vi "ColorProcessing2016_Custom.vi"(5 "LED Color Ref":refnum<vi>, 7 "Image Ctl Refnum":refnum<vi>, 9 "LED Color":T6={"Hue"={62.82225036621094, 124.95552062988281}, "Sat"={13.666671752929688, 253.6666717529297}, "Val"={150.51114654541016, 255.0}} {"Hue" scale=0.0..255.0 scale format="%#_3g"}, 10 "Mask":T5=refnum, 11 "Original":T5=refnum) -> (0 "Blob array":T2(array[cluster])=[{"Area"=410.0, "Object Info"={"Object Center"={"X"=155.50975, "Y"=158.86829}, "Bounding Box"={"X Left"=142, "Y Top"=150, "X Right"=169, "Y Bottom"=168}, "Area"=410.0, "Orientation"=9.943739, "Aspect Ratio"=1.5, "Nb Holes"=0}}], 1 "Masked":T5(plugin-control), 2 "Targets":T4[](array[typedef]), 3 "Original Image":T5(plugin-control), 4 "Scored Particle Info 2":T1(array[cluster]))   [LabVIEW 2015]
uses:
  Camera Types.ctl
  <vilib>/vision/Image Controls.llb/IMAQ Image.ctl
  Scores.ctl
  <vilib>/vision/NI_Vision_Development_Module.lvlib
panel:
  in  "Particle Count Limit":i32=3
  out "Scored Particle Info":T1(array[cluster])
  in  "Area Size Limit %":dbl=0.5
  in  "Settings":T3={"Objects"=0, "Threshold"=1, "Reject Border"=TRUE, "Fill Holes"=FALSE, "Min Object Size"=TRUE, "Min Size"=350, "Max Object Size"=TRUE, "Max Size"=700, "Show Search Area"=TRUE, "Show Center"=TRUE, "Show Bounding Box"=TRUE} {"Objects" items=["Bright Objects", "Dark Objects"]; "Threshold" min=1 max=999999999 step=1; "Max Size" min=1 max=999999999 step=1; "Min Size" min=1 max=999999999 step=1}
  out "Qualified Particles":i32=3
  out "Sorted Particle Scores":T7(array[cluster]) {"Center" format="%#_3g"; "Moment Factor" format="%#_3g"; "Aspect Ratio" format="%#_3g"; "Area to CH" format="%#_3g"; "X" format="%#_3g"; "Y" format="%#_3g"}
  out "Detected Targets":T8(array[cluster]) {"Normalized Rect"."Numeric 5" format="%#_2g"; "Normalized Rect"."Numeric 3" format="%#_2g"; "Normalized Rect"."Numeric 2" format="%#_2g"; "Normalized Rect"."Numeric" format="%#_2g"}
  in  "Aspect Ratio Fudge Factor":dbl=1.0
  out "Highest Avg Score":dbl=85.32840563115018 format="%#_3g"
  in  "Min Score Threshold":i32=70
  in  "Camera Type":T9=enum."MS HD3000 square"
  in  "Emphasize Limit Tests":bool=TRUE
  in  "Std Devs for Calibration":cluster{"H":dbl, "S":dbl, "V":dbl}={"H"=4.0, "S"=6.0, "V"=6.0}
  # "Density Profile"
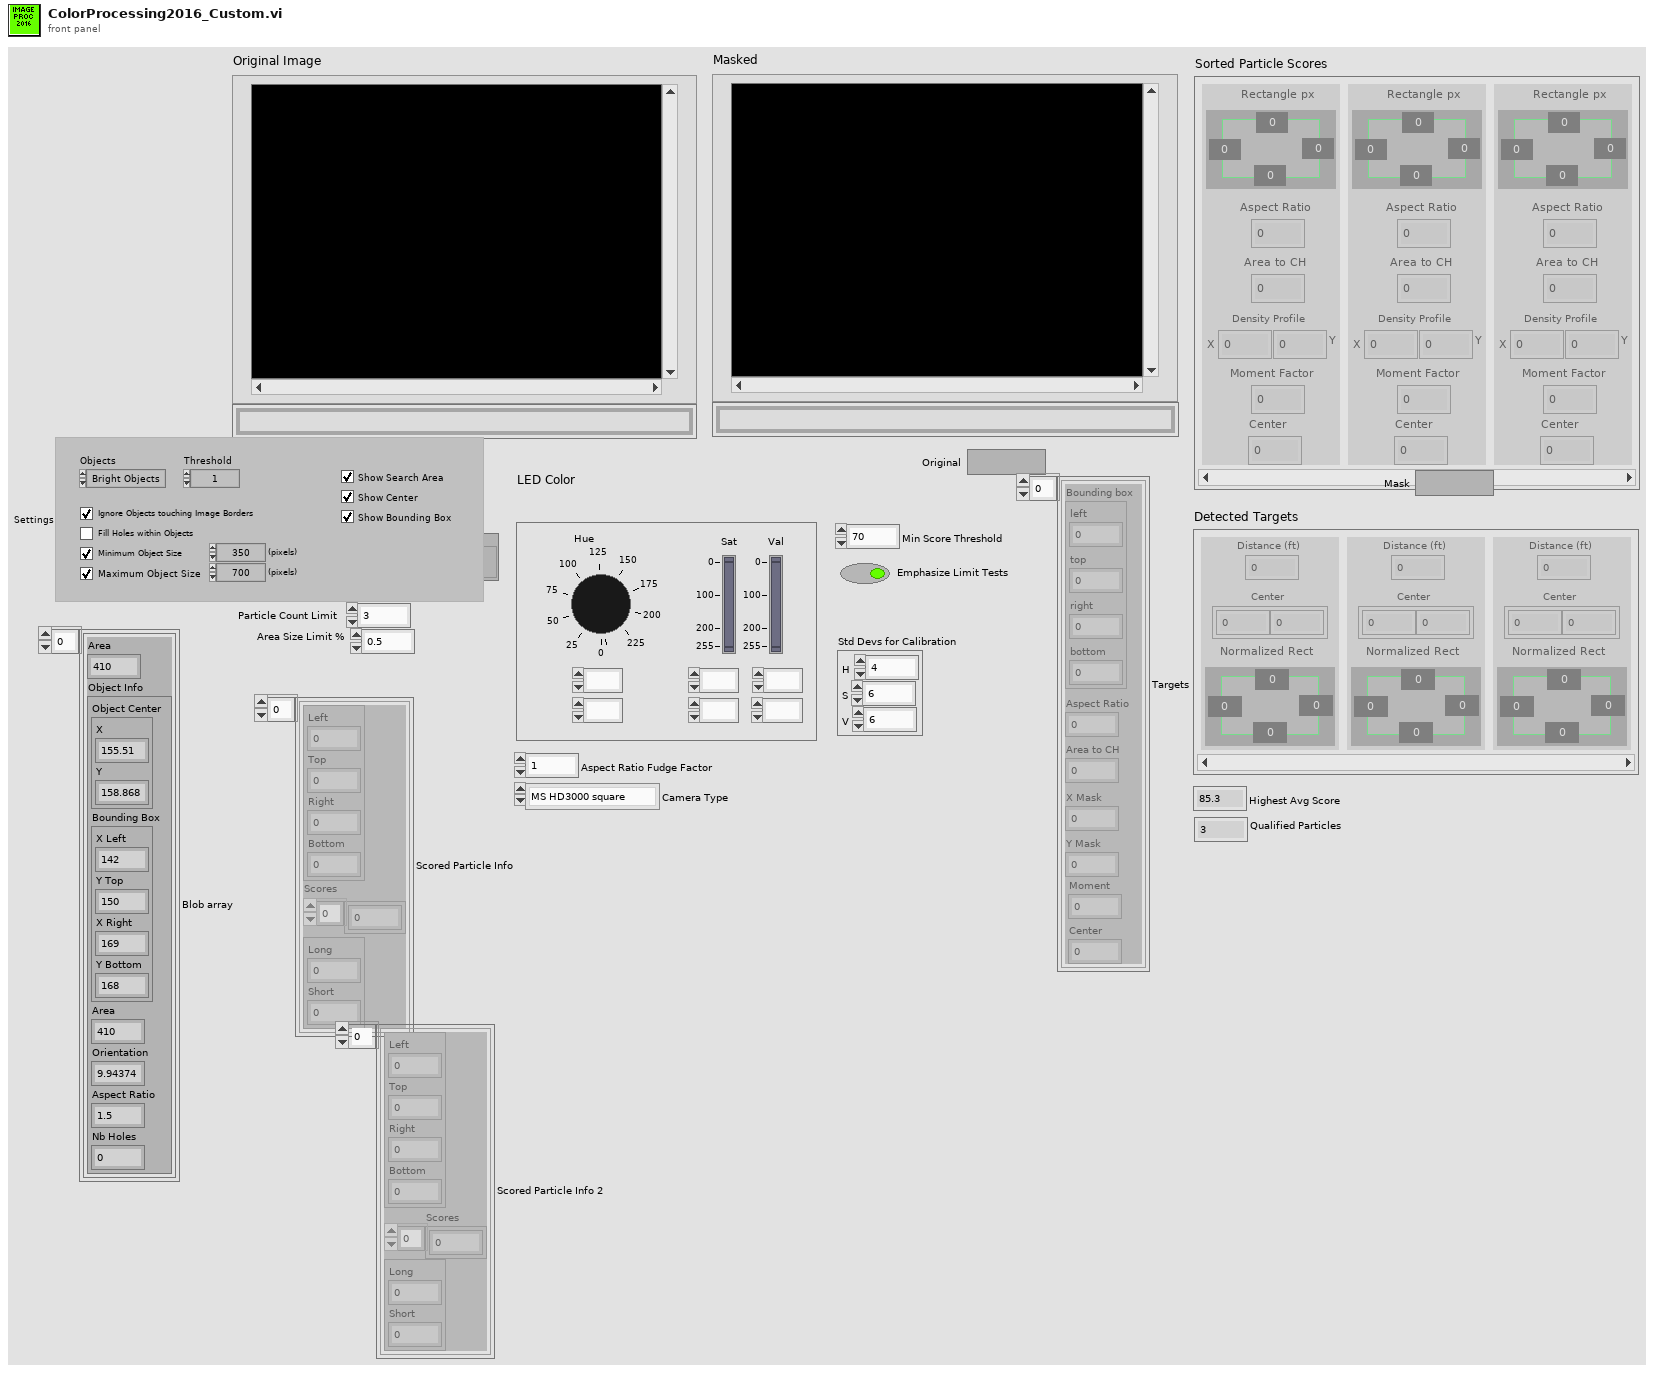
[diagram p1: front panel]
types:
  T1 = cluster{cluster{"Left":dbl, "Top":dbl, "Right":dbl, "Bottom":dbl}, "Scores":dbl[], cluster{"Long":dbl, "Short":dbl}}[]
  T2 = cluster{"Area":sgl, "Object Info":cluster{"Object Center":cluster{"X":sgl, "Y":sgl}, "Bounding Box":cluster{"X Left":i32, "Y Top":i32, "X Right":i32, "Y Bottom":i32}, "Area":sgl, "Orientation":sgl, "Aspect Ratio":sgl, "Nb Holes":i32}}[]
  T3 = cluster{"Objects":u16, "Threshold":i32, "Reject Border":bool, "Fill Holes":bool, "Min Object Size":bool, "Min Size":i32, "Max Object Size":bool, "Max Size":i32, "Show Search Area":bool, "Show Center":bool, "Show Bounding Box":bool}
  T4 = typedef "Scores.ctl" = cluster{"Bounding box":cluster{"left":dbl, "top":dbl, "right":dbl, "bottom":dbl}, "Aspect Ratio":dbl, "Area to CH":dbl, "X Mask":dbl, "Y Mask":dbl, "Moment":dbl, "Center":dbl}
  T5 = typedef "IMAQ Image.ctl" = refnum<image>
  T6 = cluster{"Hue":cluster{dbl, dbl}, "Sat":cluster{dbl, dbl}, "Val":cluster{dbl, dbl}}
  T7 = cluster{"Rectangle px":cluster{"Numeric":dbl, "Numeric 2":dbl, "Numeric 3":dbl, "Numeric 5":dbl}, "Aspect Ratio":dbl, "Area to CH":dbl, "X":dbl, "Y":dbl, "Moment Factor":dbl, "Center":dbl}[]
  T8 = cluster{"Distance (ft)":dbl, "Center":cluster{dbl, dbl}, "Normalized Rect":cluster{"Numeric":dbl, "Numeric 2":dbl, "Numeric 3":dbl, "Numeric 5":dbl}}[]
  T9 = typedef "Camera Types.ctl" = enum16{"206", "1011", "1013", "MS HD3000 square", "MS HD3000 640x480"}
  T10 = typedef "Particle Parameters" = i32
  T11 = typedef "IMAQ Rectangle" = cluster{"Left":i32, "Top":i32, "Right":i32, "Bottom":i32, "Rotation":dbl}
  T12 = typedef "Image Type" = u32
  T13 = cluster{"Object Center":cluster{"X":sgl, "Y":sgl}, "Bounding Box":cluster{"X Left":i32, "Y Top":i32, "X Right":i32, "Y Bottom":i32}, "Area":sgl, "Orientation":sgl, "Aspect Ratio":sgl, "Nb Holes":i32}[]
  T14 = cluster{"Area":sgl, "Object Info":cluster{"Object Center":cluster{"X":sgl, "Y":sgl}, "Bounding Box":cluster{"X Left":i32, "Y Top":i32, "X Right":i32, "Y Bottom":i32}, "Area":sgl, "Orientation":sgl, "Aspect Ratio":sgl, "Nb Holes":i32}}
  T15 = cluster{"Rectangle":cluster{"Numeric":dbl, "Numeric 2":dbl, "Numeric 3":dbl, "Numeric 5":dbl}, "L":dbl, "Area to CH":dbl, "X":dbl, "Y":dbl, "Moment Factor":dbl, "Center":dbl}[]
  T16 = cluster{cluster{dbl, dbl}, cluster{dbl, dbl}, cluster{dbl, dbl}}
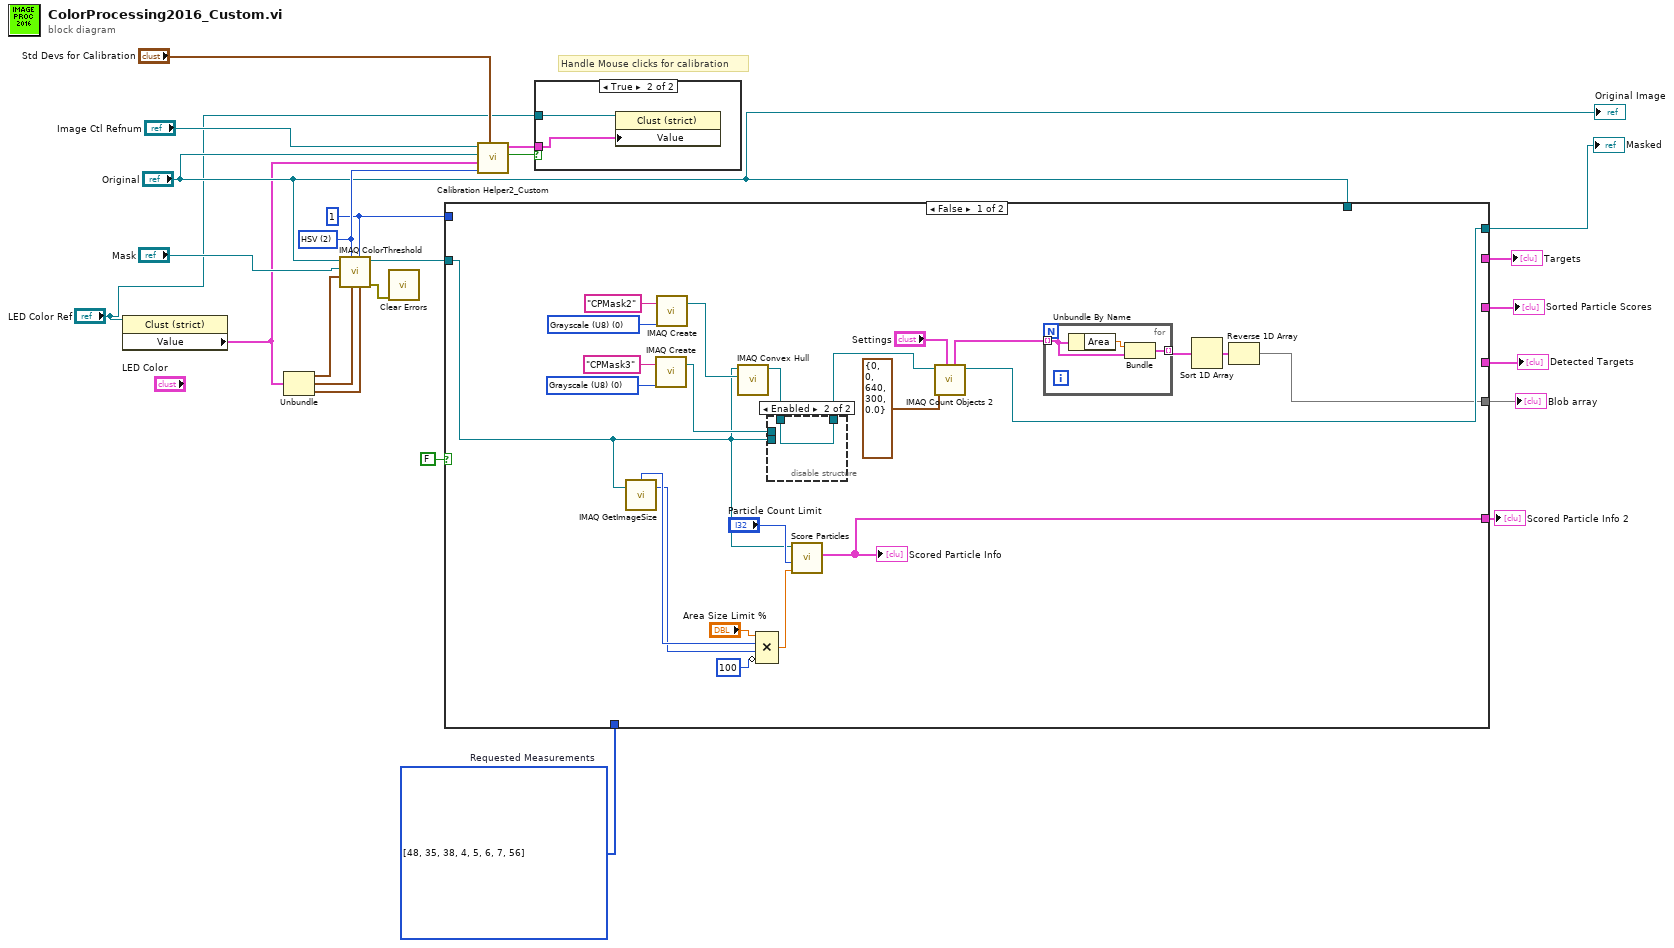
[diagram p0: block diagram]
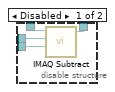
[diagram p2: hidden frame]
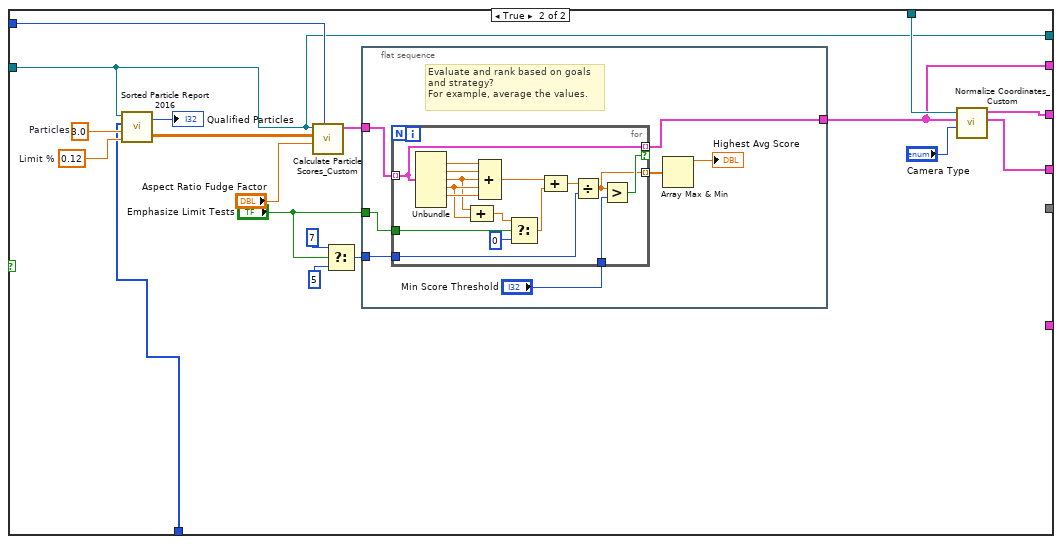
[diagram p3: hidden frame]
diagram:
  w2 = T10[] [48, 35, 38, 4, 5, 6, 7, 56] items=["Center of Mass X", "Center of Mass Y", "First Pixel X", "First Pixel Y", "Bounding Rect Left", "Bounding Rect Top", "Bounding Rect Right", "Bounding Rect Bottom", "Max Feret Diameter Start X", "Max Feret Diameter Start Y", "Max Feret Diameter End X", "Max Feret Diameter End Y", "Max Horiz. Segment Length Left", "Max Horiz. Segment Length Right", "Max Horiz. Segment Length Row", "-", "Bounding Rect Width", "Bounding Rect Height", "Bounding Rect Diagonal", "Perimeter", "Convex Hull Perimeter", "Holes' Perimeter", "Max Feret Diameter", "Equivalent Ellipse Major Axis", "Equivalent Ellipse Minor Axis", "Equivalent Ellipse Minor Axis (Feret)", "Equivalent Rect Long Side", "Equivalent Rect Short Side", "Equivalent Rect Diagonal", "Equivalent Rect Short Side (Feret)", "Average Horiz. Segment Length", "Average Vert. Segment Length", "Hydraulic Radius", "Waddel Disk Diameter", "-", "Area", "Holes' Area", "Particle & Holes' Area", "Convex Hull Area", "Image Area", "-", "Number of Holes", "Number of Horiz. Segments", "Number of Vert. Segments", "-", "Orientation", "Max Feret Diameter Orientation", "-", "% Area/Image Area", "% Area/(Particle & Holes' Area)", "Ratio of Equivalent Ellipse Axes", "Ratio of Equivalent Rect Sides", "-", "Elongation Factor", "Compactness Factor", "Heywood Circularity Factor", "Type Factor", "-", "Sum X", "Sum Y", "Sum XX", "Sum XY", "Sum YY", "Sum XXX", "Sum XXY", "Sum XYY", "Sum YYY", "-", "Moment of Inertia XX", "Moment of Inertia XY", "Moment of Inertia YY", "Moment of Inertia XXX", "Moment of Inertia XXY", "Moment of Inertia XYY", "Moment of Inertia YYY", "Norm. Moment of Inertia XX", "Norm. Moment of Inertia XY", "Norm. Moment of Inertia YY", "Norm. Moment of Inertia XXX", "Norm. Moment of Inertia XXY", "Norm. Moment of Inertia XYY", "Norm. Moment of Inertia YYY", "Hu Moment 1", "Hu Moment 2", "Hu Moment 3", "Hu Moment 4", "Hu Moment 5", "Hu Moment 6", "Hu Moment 7"]  # Requested Measurements
  w17 = 1 ("Replace Value")
  w22 = u16 2 items=["RGB", "HSL", "HSV", "HSI"] ("Color Mode")
  # "Handle Mouse clicks for calibration"
  n1 = property class="Clust (strict)"(reference="LED Color Ref") -> ("Value"=w8:T6)  [unwired: 1 in, 2 out]
  n2 = Unbundle(w8) -> ("Hue"=w14:cluster{dbl, dbl}, "Sat"=w15:cluster{dbl, dbl}, "Val"=w16:cluster{dbl, dbl})
  n3 = call "IMAQ ColorThreshold"("Blue or Luma or Val or Inten Range"=w16, "Replace Value"=w17, "Green or Sat Range"=w15, "Color Mode"=w22, "Red or Hue Range"=w14, "Image Dst"="Mask", "Image Src"="Original") -> ("error out"=w19:errorcluster, "Image Dst Out"=w6:T5)  [unwired: 3 in]
  n4 = call <vilib>:"Clear Errors.vi"("error in (no error)"=w19) -> ()  [unwired: 5 in, 2 out]
  n5 = case shown="False" FALSE {
    tunnel: [_ w65] -> w18
    tunnel: w17 -> [_ w64]
    tunnel: "Original" -> [_ w59]
    tunnel: [_ w58] -> w10
    tunnel: [_ w57] -> w9
    tunnel: w6 -> [w26 w56]
    tunnel: [w35 w56] -> w5
    tunnel: [w34 _] -> w4
    tunnel: w2 -> [_ w55]
    tunnel: [w27 _] -> w1
    frame False {
      w41 = T12 0 items=["Grayscale (U8)", "Grayscale (I16)", "Grayscale (SGL)", "Complex (CSG)", "RGB (U32)", "HSL (U32)", "RGB (U64)", "Grayscale (U16)"] ("Image Type")
      w39 = T12 0 items=["Grayscale (U8)", "Grayscale (I16)", "Grayscale (SGL)", "Complex (CSG)", "RGB (U32)", "HSL (U32)", "RGB (U64)", "Grayscale (U16)"] ("Image Type")
      n6 = call "IMAQ GetImageSize"("Image"=w26) -> ("Y Resolution"=w24:i32, "X Resolution"=w25:i32)  [unwired: 3 in, 1 out]
      n7 = call "IMAQ Create"("Image Name"="CPMask3", "Image Type"=w41) -> ("New Image"=w43:T5)  [unwired: 2 in, 2 out]
      n8 = call "IMAQ Create"("Image Name"="CPMask2", "Image Type"=w39) -> ("New Image"=w40:T5)  [unwired: 2 in, 2 out]
      n9 = call "IMAQ Convex Hull"("Image Dst"=w40, "Image Src"=w26) -> ("Image Dst Out"=w33:T5)  [unwired: 8 in, 1 out]
      n10 = Compound Arithmetic op=MULTIPLY("Area Size Limit %", w25, w24, invert 100 ("length")) -> (w28:dbl)
      n11 = disable-structure shown="Enabled" {
        disable-tunnel: w43 -> [w50 _]
        disable-tunnel: w26 -> [w49 _]
        disable-tunnel: w33 -> [w48 w51]
        disable-tunnel: [w47 w51] -> w32
        frame Disabled {
          n12 = call "IMAQ Subtract"("Image Src A"=w48, "Image Dst"=w50, "Image Src B"=w49) -> ("Image Dst Out"=w47:T5)  [unwired: 4 in, 1 out]
        }
        frame Enabled {
        }
      }
      n13 = call "Score Particles.vi"("Area Size Limit"=w28, "Particle Count Limit"="Particle Count Limit", "Image Refnum in"=w26) -> ("Scored Particle Info"=w27:T1)  [unwired: 7 in, 1 out]
      "Scored Particle Info" <- w27
      n14 = call "IMAQ Count Objects 2"("Settings"="Settings", "Search Rect (entire image)"=T11 {"Left"=0, "Top"=0, "Right"=640, "Bottom"=300, "Rotation"=0.0}, "Image"=w32) -> ("Image Out"=w35:T5, "Objects"=w44:T13)  [unwired: 4 in, 3 out]
      n15 = for {
        tunnel: w44 -> [w54] mode=indexing
        tunnel: [w52] -> w45 mode=indexing
        n16 = Unbundle By Name(w54) -> ("Area"=w53:sgl)
        n17 = Bundle("Area"=w53, "Object Info"=w54) -> (w52:T14)  [unwired: 1 in]
      }
      n18 = Sort 1D Array(array=w45) -> (sorted array=w46:T2)
      n19 = Reverse 1D Array(array=w46) -> (reversed array=w34:T2)
    }
    frame True {
      w63 = 0.12  # Limit %
      w60 = 3.0  # Particles
      n20 = call "Sorted Particle Report 2016.vi"("Min Area Size %"=w63, "Particle Count Limit"=w60, "Pixel Measurements"=w55, "Image in"=w56) -> ("Sorted Data"=w62:dbl[][], "Particles"=→"Qualified Particles":i32)
      n21 = call "Calculate Particle Scores_Custom.vi"("Pixel Value"=w64, "Aspect Fudge Factor"="Aspect Ratio Fudge Factor", "Sorted Data"=w62, "Image in"=w56) -> ("Scores"=w67:T4[])  [unwired: 7 in]
      n22 = Select(t=7, s="Emphasize Limit Tests", f=5) -> (s? t:f=w71:i32)
      n23 = flat-sequence {
        tunnel: w67 -> [w78]
        tunnel: [w79] -> w58
        tunnel: w71 -> [w75]
        tunnel: "Emphasize Limit Tests" -> [w73]
        frame #0 {
          # "Evaluate and rank based on goals\nand strategy?\nFor example, average the values."
          n24 = for {
            tunnel: w78 -> [w93] mode=indexing
            tunnel: [w93] -> w79 mode=indexing if=w92
            tunnel: [w91] -> w77 mode=indexing
            tunnel: w75 -> [w90]
            tunnel: "Min Score Threshold" -> [w89]
            tunnel: w73 -> [w82]
            n25 = Unbundle(w93) -> ("Aspect Ratio"=w95:dbl, "Area to CH"=w94:dbl, "X Mask"=w84:dbl, "Y Mask"=w85:dbl, "Moment"=w86:dbl)  [unwired: 2 out]
            n26 = Compound Arithmetic op=ADD(w84, w85) -> (w83:dbl)
            n27 = Compound Arithmetic op=ADD(w95, w94, w84, w85, w86) -> (w88:dbl)
            n28 = Select(t=w83, s=w82, f=0) -> (s? t:f=w81:dbl)
            n29 = Compound Arithmetic op=ADD(w88, w81) -> (w87:dbl)
            n30 = Divide(x=w87, y=w90) -> (x/y=w91:dbl)
            n31 = Greater?(x=w91, y=w89) -> (0:w92:bool)
          }
          n32 = Array Max & Min(array=w77) -> (max value=→"Highest Avg Score":dbl)  [unwired: 3 out]
        }
      }
      n33 = call "Normalize Coordinates_Custom.vi"("Camera Type"="Camera Type", "Targets"=w58, "Image in"=w59) -> ("Found Targets"=w65:T8, "Sorted Scores"=w57:T15)  [unwired: 7 in]
    }
  }
  "Masked" <- w5
  "Sorted Particle Scores" <- w9
  "Detected Targets" <- w18
  "Targets" <- w10
  "Blob array" <- w4
  "Scored Particle Info 2" <- w1
  n34 = call "Calibration Helper2_Custom.vi"("Std Devs"="Std Devs for Calibration", "Color Mode"=w22, "Color Components"=w8, "Image"="Original", "Image Ctl Refnum"="Image Ctl Refnum") -> ("Changed"=w20:bool, "output color"=w21:T16)  [unwired: 5 in]
  n35 = case shown="True" w20 {
    tunnel: w21 -> [_ w97]
    tunnel: "LED Color Ref" -> [_ w96]
    frame False {
    }
    frame True {
      n36 = property class="Clust (strict)"(reference=w96, "Value"=w97) -> ()  [unwired: 1 in, 2 out]
    }
  }
  "Original Image" <- "Original"
